vi "Untitled 29 (SubVI).vi"(4 "Cneg":dbl, 6 "Vneg":dbl, 7 "Vpos":dbl, 9 "y":dbl, 10 "output y(t)":dbl, 11 "Cpos":dbl) -> (3 "Numeric":dbl)   [LabVIEW 2021]
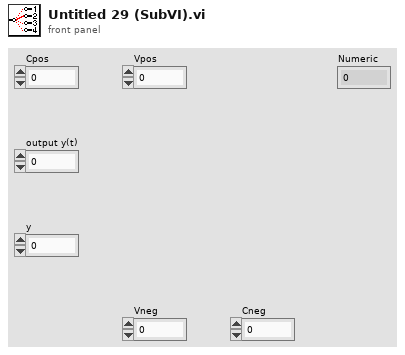
[diagram p1: front panel]
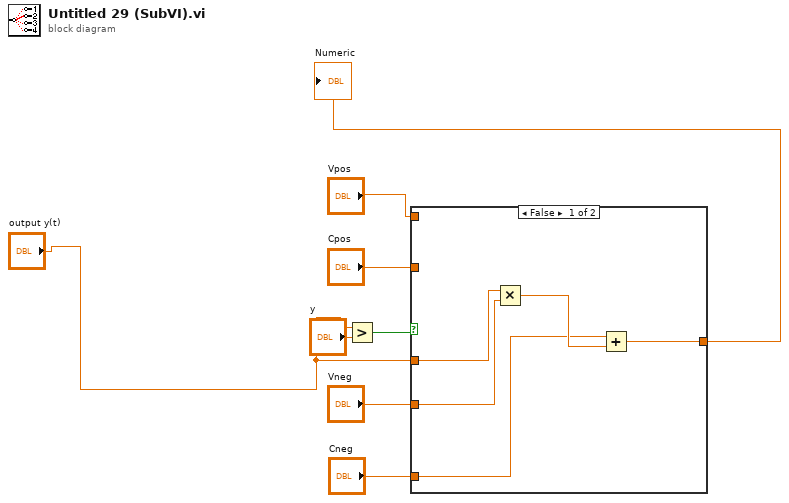
[diagram p0: block diagram]
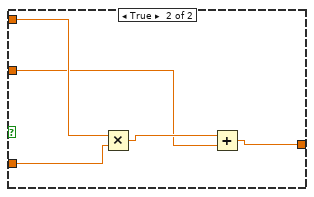
[diagram p2: hidden frame]
diagram:
  n1 = Greater?(x="output y(t)", y="y") -> (0:w2:bool)
  n2 = case shown="False" w2 {
    tunnel: [w9 w14] -> w1
    tunnel: "Vpos" -> [_ w18]
    tunnel: "output y(t)" -> [w10 w17]
    tunnel: "Cpos" -> [_ w15]
    tunnel: "Cneg" -> [w12 _]
    tunnel: "Vneg" -> [w11 _]
    frame False {
      n3 = Multiply ("Multiply 2")(x=w10, y=w11) -> (x*y=w13:dbl)
      n4 = Add ("Add 2")(x=w12, y=w13) -> (x+y=w9:dbl)
    }
    frame True {
      n5 = Multiply(x=w18, y=w17) -> (x*y=w16:dbl)
      n6 = Add(x=w16, y=w15) -> (x+y=w14:dbl)
    }
  }
  "Numeric" <- w1
